vi "PEAK_Init.vi"(8 "errin":errorcluster) -> (0 "errout":errorcluster, 3 "Channel out":T1)   [LabVIEW 2020, in "PEAK_lib_ALEX.lvlib"]
uses:
  PEAK_lib_ALEX.lvlib
  PCAN Basic/Controls/Channel.ctl
  PCAN Basic/Controls/Parameter.ctl
  PCAN Basic/Controls/BaudrateEenum.ctl
  PCAN Basic/VIs/Get Value/PCAN Get CHANNEL CONDITION.vi
  PCAN Basic/PCANBasic.lvlib
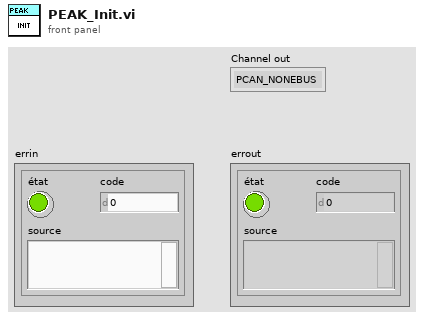
[diagram p1: front panel]
types:
  T1 = typedef "PCANBasic.lvlib/Channel.ctl" = enum16{"PCAN_NONEBUS", "not used1", "not used2", "not used3", "not used4", "not used5", "not used6", "not used7", "not used8", "not used9", "not used10", "not used11", "not used12", "not used13", "not used14", "not used15", "not used16", "not used17", "not used18", "not used19", "not used20", "not used21", "not used22", "not used23", "not used24", "not used25", "not used26", "not used27", "not used28", "not used29", "not used30", "not used31", "not used32", "PCAN_ISABUS1", "PCAN_ISABUS2", "PCAN_ISABUS3", "PCAN_ISABUS4", "PCAN_ISABUS5", "PCAN_ISABUS6", "PCAN_ISABUS7", "PCAN_ISABUS8", "not used41", "not used42", "not used43", "not used44", "not used45", "not used46", "not used47", "not used48", "PCAN_DNGBUS1", "not used50", "not used51", "not used52", "not used53", "not used54", "not used55", "not used56", "not used57", "not used58", "not used59", "not used60", "not used61", "not used62", "not used63", "not used64", "PCAN_PCIBUS1", "PCAN_PCIBUS2", "PCAN_PCIBUS3", "PCAN_PCIBUS4", "PCAN_PCIBUS5", "PCAN_PCIBUS6", "PCAN_PCIBUS7", "PCAN_PCIBUS8", "not used73", "not used74", "not used75", "not used76", "not used77", "not used78", "not used79", "not used80", "PCAN_USBBUS1", "PCAN_USBBUS2", "PCAN_USBBUS3", "PCAN_USBBUS4", "PCAN_USBBUS5", "PCAN_USBBUS6", "PCAN_USBBUS7", "PCAN_USBBUS8", "Not used89", "Not used90", "Not used91", "Not used92", "Not used93", "Not used94", "Not used95", "Not used96", "PCAN_PCCBUS1", "PCAN_PCCBUS2"}
  T2 = typedef "PCANBasic.lvlib/BaudrateEenum.ctl" = enum16{"CAN_Baud_1M", "CAN_Baud_800K", "CAN_BAUD_500K", "CAN_BAUD_250K", "CAN_BAUD_125K", "CAN_BAUD_100K", "CAN_BAUD_95K", "CAN_BAUD_83K", "CAN_BAUD_50K", "CAN_BAUD_47K", "CAN_BAUD_33K", "CAN_BAUD_20K", "CAN_BAUD_10K", "CAN_BAUD_5K", "User Baudrate"}
  T3 = typedef "PCANBasic.lvlib/Parameter.ctl" = enum16{"Not Available", "PCAN device number", "PCAN 5-volt power", "PCAN receive event", "PCAN message filter", "PCAN API version", "PCAN channel version", "PCAN bus-off auto reset", "PCAN listen-only", "PCAN log location", "PCAN log status", "PCAN log configure", "PCAN log text", "PCAN channel condition", "PCAN hardware name"}
  T4 = typedef "PCANBasic.lvlib/Channel Availability.ctl" = enum16{"PCAN_CHANNEL_UNAVAILABLE", "PCAN_CHANNEL_AVAILABLE ", "PCAN_CHANNEL_OCCUPIED "}
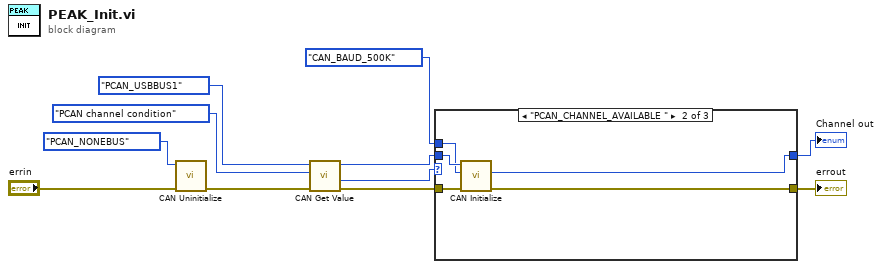
[diagram p0: block diagram]
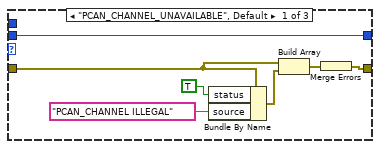
[diagram p2: hidden frame]
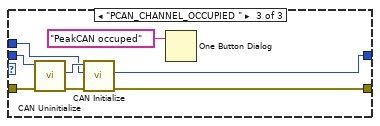
[diagram p3: hidden frame]
diagram:
  n1 = call "CAN Uninitialize.vi"("error in (no error)"="errin", "Channel"=Channel."PCAN_NONEBUS") -> ("error out"=w4:errorcluster)  [unwired: 7 in, 2 out]
  n2 = call-poly "CAN Get Value.vi"("error in (no error)"=w4, "Parameter"=Parameter."PCAN channel condition", "Channel"=Channel."PCAN_USBBUS1") -> ("error out"=w6:errorcluster, "Channel condition"=w8:T4, "Channel out"=w7:T1)  [unwired: 6 in]
  n3 = case shown="\"PCAN_CHANNEL_AVAILABLE \"" w8 {
    tunnel: [w17 w23 w26] -> w11
    tunnel: w7 -> [w18 w22 w30]
    tunnel: w6 -> [w16 w21 w31]
    tunnel: BaudrateEenum."CAN_BAUD_500K" ("BTR0BTR1") -> [_ w20 w27]
    tunnel: [w18 w19 w25] -> w10
    frame "PCAN_CHANNEL_UNAVAILABLE", Default {
      n4 = Bundle By Name(cluster=w16, "status"=TRUE, "source"="PCAN_CHANNEL ILLEGAL") -> (w13:errorcluster)
      n5 = Build Array(w16, w13) -> (w12:errorcluster[])
      n6 = Merge Errors(w12) -> (w17:errorcluster)
    }
    frame "PCAN_CHANNEL_AVAILABLE " {
      n7 = call "CAN Initialize.vi"("error in (no error)"=w21, "BTR0BTR1"=w20, "Channel"=w22) -> ("error out"=w23:errorcluster, "Channel out"=w19:T1)  [unwired: 6 in, 1 out]
    }
    frame "PCAN_CHANNEL_OCCUPIED " {
      n8 = call "CAN Uninitialize.vi"("error in (no error)"=w31, "Channel"=w30) -> ("error out"=w29:errorcluster, "Channel out"=w28:T1)  [unwired: 7 in, 1 out]
      n9 = call "CAN Initialize.vi"("error in (no error)"=w29, "BTR0BTR1"=w27, "Channel"=w28) -> ("error out"=w26:errorcluster, "Channel out"=w25:T1)  [unwired: 6 in, 1 out]
      n10 = One Button Dialog(message="PeakCAN occuped") -> ()  [unwired: 1 in, 1 out]
    }
  }
  "errout" <- w11
  "Channel out" <- w10
